vi "DHT11Measurement.vi"(0 "Serial Name":string="ASRL1::INSTR", 1 "Perform Measurement":bool, 2 "baud rate":u32=9600, 3 "Delay [ms]":dbl=0.01 format="%#_13g", 5 "Error In":errorcluster) -> (6 "Temperature (C)":dbl, 7 "Humidity (%)":dbl, 8 "error out":errorcluster)   [LabVIEW 2017]
doc: "Todo"
uses:
  <vilib>/Instr/_visa.llb/VISA Configure Serial Port (Instr).vi
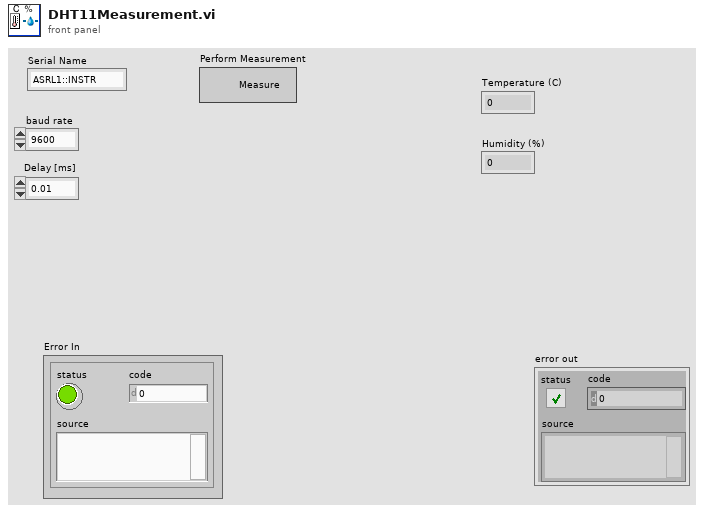
[diagram p1: front panel]
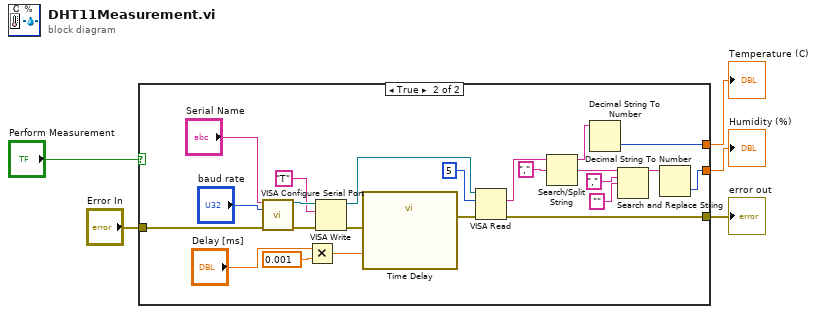
[diagram p0: block diagram]
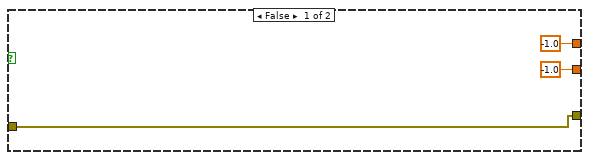
[diagram p2: hidden frame]
diagram:
  n1 = case shown="True" "Perform Measurement" {
    tunnel: "Error In" -> [w8 w12]
    tunnel: [w8 w11] -> w4
    tunnel: [-1.0 w10] -> w2
    tunnel: [-1.0 w9] -> w1
    frame False {
    }
    frame True {
      n2 = call-poly "VISA Configure Serial Port"("VISA resource name"="Serial Name", "baud rate (9600)"="baud rate", "error in (no error)"=w12) -> ("VISA resource name out"=w30:refnum<visa-resource-name>, "error out"=w31:errorcluster)  [unwired: 11 in]
      n3 = Multiply(x="Delay [ms]", y=0.001) -> (x*y=w14:dbl)
      n4 = VISA Write(VISA resource name=w30, write buffer="T", error in (no error)=w31) -> (VISA resource name out=w23:refnum<visa-resource-name>, error out=w28:errorcluster)  [unwired: 1 out]
      n5 = call "Time Delay"("error in (no error)"=w28, "Delay Time (s)"=w14) -> ("error out"=w29:errorcluster)  [unwired: 9 in]
      n6 = VISA Read(VISA resource name=w23, byte count=5, error in (no error)=w29) -> (read buffer=w24:string, error out=w11:errorcluster)  [unwired: 2 out]
      n7 = Search/Split String(string=w24, search string/char (-)=",") -> (substring before match=w25:string, match + rest of string=w26:string)  [unwired: 1 in, 1 out]
      n8 = Decimal String To Number(string=w25) -> (number=w10:i32)  [unwired: 2 in, 1 out]
      n9 = Search and Replace String(input string=w26, search string=",", replace string="") -> (result string=w27:string)  [unwired: 5 in, 3 out]
      n10 = Decimal String To Number(string=w27) -> (number=w9:i32)  [unwired: 2 in, 1 out]
    }
  }
  "error out" <- w4
  "Temperature (C)" <- w2
  "Humidity (%)" <- w1
